vi "FFT Spectrum (Mag-Phase) for 1 Chan.vi"(4 "window parameter":dbl=nan, 6 "averaging parameters":T2={"averaging mode"=enum."No averaging", "weighting mode"=enum."Exponential", "number of averages"=10} {"number of averages" min=1}, 7 "restart averaging (F)":bool, 8 "error in (no error)":errorcluster, 9 "view":T1, 10 "window":T3=1 items=["Rectangle"=0, "Hanning"=1, "Hamming"=2, "Blackman-Harris"=3, "Exact Blackman"=4, "Blackman"=5, "Flat Top"=6, "4 Term B-Harris "=7, "7 Term B-Harris"=8, "Low Sidelobe"=9, "Blackman Nuttall"=11, "Triangle"=30, "Bartlett-Hanning"=31, "Bohman"=32, "Parzen"=33, "Welch"=34, "Kaiser"=60, "Dolph-Chebyshev"=61, "Gaussian"=62], 11 "time signal":waveform(dbl)) -> (0 "error out":errorcluster, 1 "averages completed":dbl, 2 "phase":cluster{"f0":dbl, "df":dbl, "phase":dbl[]} {"phase" format="%.2p"; "f0" format="%0.2p"; "df" format="%0.2p"}, 3 "magnitude":cluster{"f0":dbl, "df":dbl, "magnitude":dbl[]} {"magnitude" format="%.2p"; "f0" format="%0.2p"; "df" format="%0.2p"}, 5 "averaging done":bool)   [LabVIEW 2020, in "NI_MAPro.lvlib"]
doc: "Computes the averaged FFT spectrum of <B>time signal</B>. This VI returns the FFT results as <B>magnitude</B> and <B>phase</B>. Wire data to the <B>time signal</B> input to determine the polymorphic instance to use or manually select the instance."
uses:
  NI_MAPro.lvlib
  windowTd.ctl
  NI_AALPro.lvlib
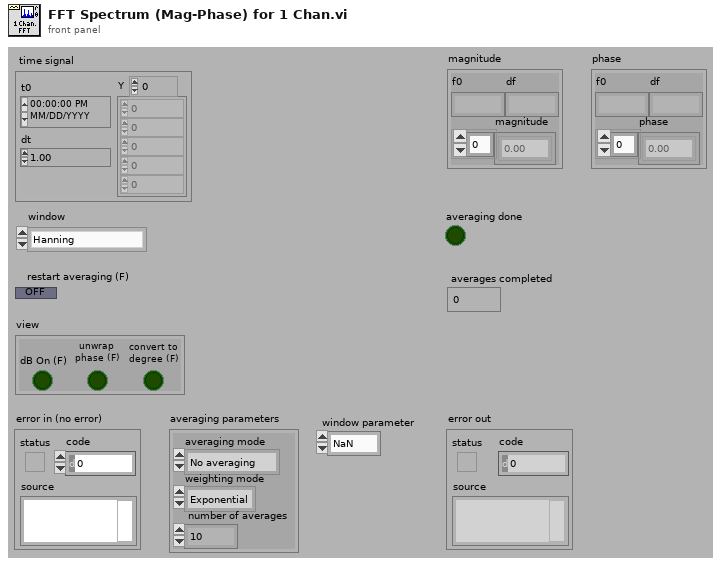
[diagram p1: front panel]
types:
  T1 = cluster{"dB On (F)":bool, "unwrap phase (F)":bool, "convert to degree (F)":bool}
  T2 = cluster{"averaging mode":enum16{"No averaging", "Vector averaging", "RMS averaging", "Peak hold"}, "weighting mode":enum16{"Linear", "Exponential"}, "number of averages":u32}
  T3 = typedef "NI_AALPro.lvlib/windowTd.ctl" = u32
  T4 = cluster{"block size":i32, "dt":dbl, "spectrum parameters":cluster{"averaging parameters":cluster{"averaging mode":enum16{"No averaging", "Vector averaging", "RMS averaging", "Peak hold"}, "weighting mode":enum16{"Linear", "Exponential"}, "number of averages":u32}, "window":T3}, "df":dbl, "averages completed":dbl, "complex spectrum":cdb[], "real spectrum":dbl[], "t0 history":dbl, "dt history":dbl, "timestamp":dbl, "lin avg done":bool}
  T5 = cluster{"f0":dbl, "df":dbl, "imag or phase":dbl[]}
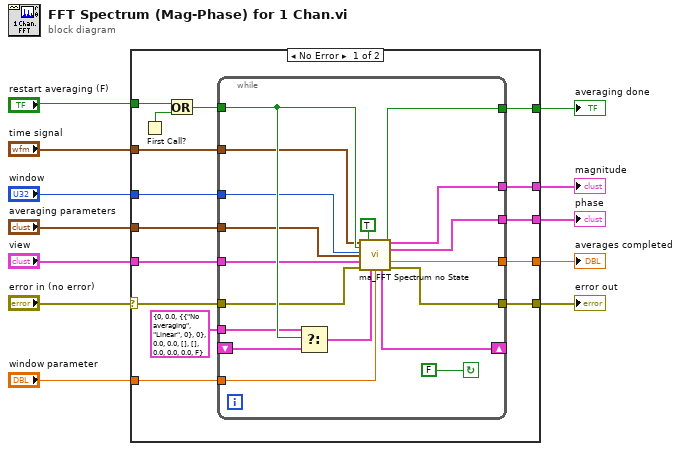
[diagram p0: block diagram]
diagram:
  n1 = case shown="No Error" "error in (no error)" {
    selector: "error in (no error)" -> [w24 w46]
    tunnel: [w25 w46] -> w12
    tunnel: "restart averaging (F)" -> [w22 _]
    tunnel: "time signal" -> [w21 _]
    tunnel: "window" -> [w20 _]
    tunnel: "averaging parameters" -> [w19 _]
    tunnel: "view" -> [w18 _]
    tunnel: "window parameter" -> [w17 _]
    tunnel: [w16 _] -> w4
    tunnel: [w15 _] -> w3
    tunnel: [w14 _] -> w2
    tunnel: [w13 _] -> w1
    frame No Error {
      n2 = First Call?() -> (First Call?: T/F=w27:bool)
      n3 = Or(x=w22, y=w27) -> (x .or. y?=w26:bool)
      n4 = while {
        tunnel: w20 -> [w37]
        tunnel: w24 -> [w38]
        tunnel: w21 -> [w36]
        tunnel: w19 -> [w35]
        tunnel: w26 -> [w40]
        tunnel: [w45] -> w13
        tunnel: [w44] -> w16
        tunnel: [w43] -> w14
        tunnel: [w42] -> w25
        shift-right: [w41] -> _
        shift-left: _ -> [w32]
        tunnel: T4 {"block size"=0, "dt"=0.0, "spectrum parameters"={"averaging parameters"={"averaging mode"=enum."No averaging", "weighting mode"=enum."Linear", "number of averages"=0}, "window"=0}, "df"=0.0, "averages completed"=0.0, "complex spectrum"=[], "real spectrum"=[], "t0 history"=0.0, "dt history"=0.0, "timestamp"=0.0, "lin avg done"=FALSE} ("state info") -> [w39]
        tunnel: w18 -> [w31]
        tunnel: [w29] -> w15
        tunnel: w17 -> [w28]
        stop <- FALSE continue-if-true
        n5 = Select(t=w39, s=w40, f=w32) -> (s? t:f=w33:T4)
        n6 = call "ma_FFT Spectrum no State.vi"("time signal"=w36, "restart averaging (F)"=w40, "mag-phase"=TRUE, "window"=w37, "averaging parameters"=w35, "view"=w31, "error in"=w38, "state info"=w33, "window parameter"=w28) -> ("averaging done"=w45:bool, "real or mag"=w43:cluster{"f0":dbl, "df":dbl, "real or mag":dbl[]}, "imag or phase"=w29:T5, "averages completed"=w44:dbl, "state info"=w41:T4, "error out"=w42:errorcluster)  [unwired: 1 out]
      }
    }
    frame Error {
    }
  }
  "error out" <- w12
  "averages completed" <- w4
  "averaging done" <- w1
  "phase" <- w3
  "magnitude" <- w2
